vi "PH_TKTDS-30xx.set Trigger GUI Element.vi"(2 "Ref Trigger Config":refnum<vi>, 3 "Trigger Config":T1={"Source"="CH1", "Slope"=0, "Level [V]"=0.0} {"Level [V]" format="%#_6p"}, 5 "error in":errorcluster) -> (19 "error out":errorcluster)   [LabVIEW 2014, in "PH_TKTDS-30xx.lvlib"]
doc: "If the reference is valid, the incoming data are set to the GUI."
uses:
  PH_TKTDS-30xx.lvlib
  PH_TKTDS-30xx.Trigger Config.ctl
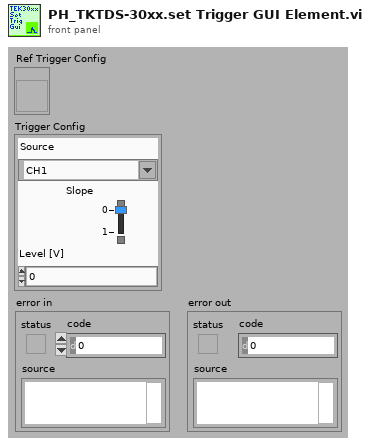
[diagram p1: front panel]
types:
  T1 = typedef "PH_TKTDS-30xx.lvlib/PH_TKTDS-30xx.Trigger Config.ctl" = cluster{"Source":string, "Slope":i32, "Level [V]":dbl}
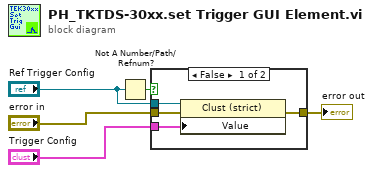
[diagram p0: block diagram]
diagram:
  n1 = Not A Number/Path/Refnum?(number/path/refnum="Ref Trigger Config") -> (NaN/Path/Refnum?=w5:bool)
  n2 = case shown="False" w5 {
    tunnel: "error in" -> [w9 w10]
    tunnel: [w8 w10] -> w3
    tunnel: "Ref Trigger Config" -> [w7 _]
    tunnel: "Trigger Config" -> [w6 _]
    frame False {
      n3 = property class="Clust (strict)"(reference=w7, error in=w9, "Value"=w6) -> (error out=w8:errorcluster)  [unwired: 1 out]
    }
    frame True {
    }
  }
  "error out" <- w3
